vi "picoharp_write_action_for_records.vi"(8 "error in (no error)":errorcluster, 10 "action_for_records":T1, 11 "hydraharp in":refnum<class "picoharp.lvclass">) -> (0 "error out":errorcluster, 3 "hydraharp out":refnum<class "picoharp.lvclass">)   [LabVIEW 2015, in "picoharp.lvclass"]
uses:
  picoharp.lvclass
  Hydraharp/hydraharp/hydraharp_action_on_records.ctl
  picoharp.lvclass/picoharp.ctl
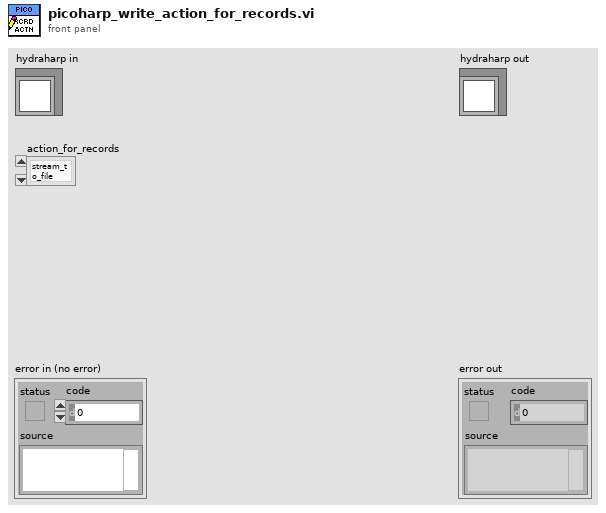
[diagram p1: front panel]
types:
  T1 = typedef "hydraharp_action_on_records.ctl" = enum16{"stream_to_file", "correlate", "stream to file and correlate"}
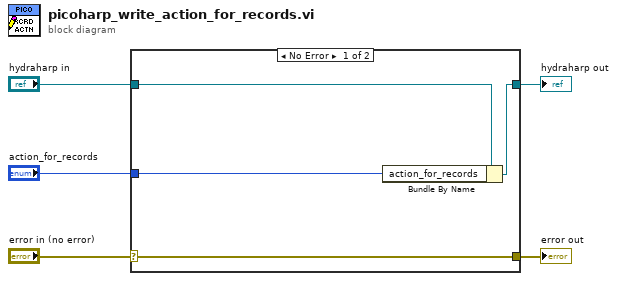
[diagram p0: block diagram]
diagram:
  n1 = case shown="No Error" "error in (no error)" {
    selector: "error in (no error)" -> [w9 w10]
    tunnel: [w9 w10] -> w4
    tunnel: [w7 w11] -> w2
    tunnel: "hydraharp in" -> [w8 w11]
    tunnel: "action_for_records" -> [w6 _]
    frame No Error {
      n2 = Bundle By Name(cluster=w8, "action_for_records"=w6) -> (w7:refnum<class "picoharp.lvclass">)
    }
    frame Error {
    }
  }
  "error out" <- w4
  "hydraharp out" <- w2
